vi "Master_DAQ.vi"(8 "error in (no error)":errorcluster) -> (0 "error out":errorcluster)   [LabVIEW 2018]
doc: "Reads actual data from inputs or virtual data for testing. Converts the data into an array of double precision values and sends it to the user, HostMain.vi, and the main control loop."
uses:
  Type_Def/TypeDef_LoopPeriod.ctl
  Type_Def/Type_Def NetworkStreamState.ctl
  Type_Def/Master_DataControl.ctl
  Type_Def/TypeDef_cRIODatas.ctl
  Type_Def/Type_Def IMUDatas.ctl
  Type_Def/TypeDef_BMSDatas.ctl
  Type_Def/TypeDef_BMSStatuss.ctl
  Type_Def/TypeDef FixedMotorData.ctl
  Type_Def/Type_Def Master_DataControls.ctl
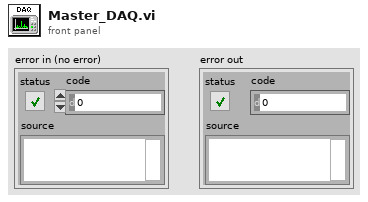
[diagram p1: front panel]
types:
  T1 = typedef "TypeDef_LoopPeriod.ctl" = cluster{"Control Period":i64, "DAQ Period":u32, "IMU Period":u32, "CAN Period":i64, "Nav Period":u32}
  T2 = typedef "Type_Def NetworkStreamState.ctl" = enum16{"Wait", "Test", "Initialize", "Read/Write", "Terminate"}
  T3 = typedef "Type_Def Master_DataControls.ctl" = cluster{"cRIO Data":T4, "IMU Data":T5, "BMS Data":T6, "Motor Data":T8}
  T4 = typedef "TypeDef_cRIODatas.ctl" = cluster{"HallEffect Right (cm)":dbl, "HallEffect Left (cm)":dbl, "Optical Sensor 1 (V)":dbl, "Optical Sensor 2 (V)":dbl, "24V Voltage  (V)":dbl, "24V Current (A)":dbl, "Contactor H1 Continuity":dbl, "Contactor L1 Continuity ":dbl, "Contactor H2 Continuity":dbl, "Contactor L2 Continuity ":dbl, "Brake PT(psig)":dbl, "Pump PT (psig)":dbl, "24V Temp   (C)":dbl, "Tank PT(psig) ":dbl, "ABS Pressure 1 (psig)":dbl, "ABS Pressure 2 (psig) ":dbl, "Displacement (ft)":dbl, "Velocity (ft/s)":dbl, "Time (ms)":dbl}
  T5 = typedef "Type_Def IMUDatas.ctl" = cluster{"x acceleration (g)":dbl, "Pressure (psia)":dbl, "Temperature (F)":dbl}
  T6 = typedef "TypeDef_BMSDatas.ctl" = cluster{"Pack 1 Max Cell\n Voltage (V)":dbl, "Pack 1 Max Cell\n ID ":dbl, "Pack 1 Min Cell \nVoltage (V)":dbl, "Pack 1 Min Cell \nID ":dbl, "Pack 1 State of Charge  (%)":dbl, "Pack 1 Average Voltage1 (V)":dbl, "Pack 1Voltage Delta (V)":dbl, "Pack 1 Current (A)":dbl, "Pack 1 Voltage (V)":dbl, "Pack 1 Max Resistance (Ohm)":dbl, "Pack 1Min Resistance (Ohm)":dbl, "Pack 1Average Resistance (Ohm)":dbl, "Pack 1Delta Resistance (Ohm)":dbl, "Pack 1 Highest Temperature(F)":dbl, "BmsStatus":T7, "Pack 2 Max Cell\n Voltage (V) ":dbl, "Pack 2 Max Cell\n ID  ":dbl, "Pack 2 Min Cell \nVoltage (V) ":dbl, "Pack 2 Min Cell \nID  ":dbl, "Pack 2 Average Voltage1 (V)":dbl, "Pack 2 Voltage Delta (V) ":dbl, "Pack 2 Current (A)":dbl, "Pack 2 Voltage (V) ":dbl, "Pack 2 State of Charge  (%) ":dbl, "Pack 2 Max Resistance (Ohm) ":dbl, "Pack 2 Min Resistance (Ohm)":dbl, "Pack 2 Average Resistance (Ohm)":dbl, "Pack 2 Delta Resistance (Ohm) ":dbl, "Pack 2 Highest Temperature(F) ":dbl}
  T7 = typedef "TypeDef_BMSStatuss.ctl" = cluster{"isFault":bool, "isolationMonitoring":bool, "isFault 2":bool, "isolationMonitoring 2":bool}
  T8 = typedef "TypeDef FixedMotorData.ctl" = cluster{" Velocity (RPM)":dbl, " MotorTemp(C)":dbl, " ControlTemp(C)":dbl, " DcLinkVolt(V)":dbl, " ErrorCode":dbl, "IsAlive":bool, "motorStatus":cluster{"isReady":bool, "isOn":bool, "isOperEn":bool, "isFault":bool, "isVoltEn":bool, "targetReached":bool, "isWarning":bool}, "motorControllerState":u16}
  T9 = typedef "Master_DataControl.ctl" = cluster{"cRIO Data":T4, "IMU Data":T5, "BMS Data":T6, "Motor Data":T8}
  T10 = cluster{"x acceleration (g)":dbl, "Pressure (psia)":dbl, "Temperature (F)":dbl}
  T11 = typedef "TypeDef_NetworkStreamState.ctl" = enum16{"Wait", "Test", "Initialize", "Read/Write", "Terminate"}
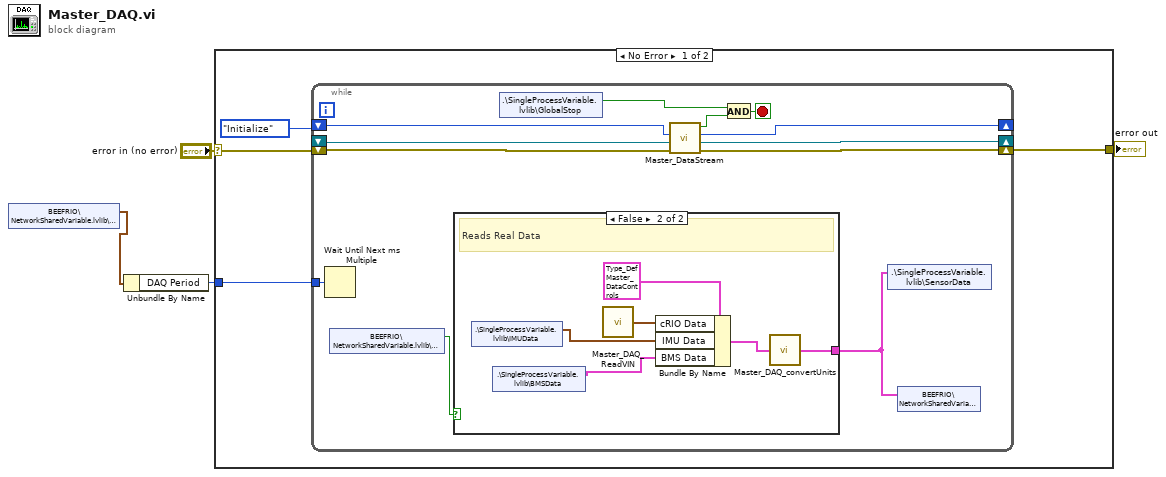
[diagram p0: block diagram]
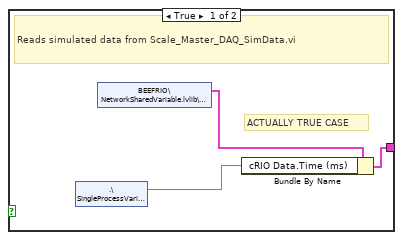
[diagram p2: hidden frame]
diagram:
  n1 = shared-variable "BEEFRIO\\NetworkSharedVariable.lvlib\\LoopPeriods"() -> (w1:T1)  [unwired: 1 in, 1 out]
  n2 = Unbundle By Name(w1) -> ("DAQ Period"=w2:u32)
  n3 = case shown="No Error" "error in (no error)" {
    selector: "error in (no error)" -> [w8 w30]
    tunnel: [w7 w30] -> w3
    tunnel: w2 -> [w6 _]
    frame No Error {
      n4 = while {
        shift-right: [w16] -> w7
        shift-left: w8 -> [w17]
        shift-right: [w20] -> _
        shift-left: _ -> [w14]
        tunnel: w6 -> [w15]
        shift-right: [w9] -> _
        shift-left: Type_Def_NetworkStreamState."Initialize" ("Enum") -> [w10]
        stop <- w19 stop-if-true
        n5 = Wait Until Next ms Multiple(millisecond multiple=w15) -> ()  [unwired: 1 out]
        n6 = shared-variable "BEEFRIO\\NetworkSharedVariable.lvlib\\SimulateData"() -> (w11:bool)  [unwired: 1 in, 1 out]
        n7 = case shown="False" w11 {
          tunnel: [w21 w24] -> w12
          frame True {
            # "ACTUALLY TRUE CASE"
            # "Reads simulated data from Scale_Master_DAQ_SimData.vi"
            n8 = shared-variable ".\\SingleProcessVariable.lvlib\\Time"() -> (w23:dbl)  [unwired: 1 in, 1 out]
            n9 = shared-variable "BEEFRIO\\NetworkSharedVariable.lvlib\\DataOverride"() -> (w22:T9)  [unwired: 1 in, 1 out]
            n10 = Bundle By Name(cluster=w22, "cRIO Data.Time (ms)"=w23) -> (w21:T9)
          }
          frame False {
            # "Reads Real Data"
            n11 = shared-variable ".\\SingleProcessVariable.lvlib\\IMUData"() -> (w26:T10)  [unwired: 1 in, 1 out]
            n12 = shared-variable ".\\SingleProcessVariable.lvlib\\BMSData"() -> (w25:T6)  [unwired: 1 in, 1 out]
            n13 = call "Master_DAQ_ReadVIN.vi"() -> ("cRIO Data"=w27:T4)  [unwired: 1 in]
            n14 = Bundle By Name(cluster=T3 {"cRIO Data"={"HallEffect Right (cm)"=0.0, "HallEffect Left (cm)"=0.0, "Optical Sensor 1 (V)"=0.0, "Optical Sensor 2 (V)"=0.0, "24V Voltage  (V)"=0.0, "24V Current (A)"=0.0, "Contactor H1 Continuity"=0.0, "Contactor L1 Continuity "=0.0, "Contactor H2 Continuity"=0.0, "Contactor L2 Continuity "=0.0, "Brake PT(psig)"=0.0, "Pump PT (psig)"=0.0, "24V Temp   (C)"=0.0, "Tank PT(psig) "=0.0, "ABS Pressure 1 (psig)"=0.0, "ABS Pressure 2 (psig) "=0.0, "Displacement (ft)"=0.0, "Velocity (ft/s)"=0.0, "Time (ms)"=0.0}, "IMU Data"={"x acceleration (g)"=0.0, "Pressure (psia)"=0.0, "Temperature (F)"=0.0}, "BMS Data"={"Pack 1 Max Cell\n Voltage (V)"=0.0, "Pack 1 Max Cell\n ID "=0.0, "Pack 1 Min Cell \nVoltage (V)"=0.0, "Pack 1 Min Cell \nID "=0.0, "Pack 1 State of Charge  (%)"=0.0, "Pack 1 Average Voltage1 (V)"=0.0, "Pack 1Voltage Delta (V)"=0.0, "Pack 1 Current (A)"=0.0, "Pack 1 Voltage (V)"=0.0, "Pack 1 Max Resistance (Ohm)"=0.0, "Pack 1Min Resistance (Ohm)"=0.0, "Pack 1Average Resistance (Ohm)"=0.0, "Pack 1Delta Resistance (Ohm)"=0.0, "Pack 1 Highest Temperature(F)"=0.0, "BmsStatus"={"isFault"=FALSE, "isolationMonitoring"=FALSE, "isFault 2"=FALSE, "isolationMonitoring 2"=FALSE}, "Pack 2 Max Cell\n Voltage (V) "=0.0, "Pack 2 Max Cell\n ID  "=0.0, "Pack 2 Min Cell \nVoltage (V) "=0.0, "Pack 2 Min Cell \nID  "=0.0, "Pack 2 Average Voltage1 (V)"=0.0, "Pack 2 Voltage Delta (V) "=0.0, "Pack 2 Current (A)"=0.0, "Pack 2 Voltage (V) "=0.0, "Pack 2 State of Charge  (%) "=0.0, "Pack 2 Max Resistance (Ohm) "=0.0, "Pack 2 Min Resistance (Ohm)"=0.0, "Pack 2 Average Resistance (Ohm)"=0.0, "Pack 2 Delta Resistance (Ohm) "=0.0, "Pack 2 Highest Temperature(F) "=0.0}, "Motor Data"={" Velocity (RPM)"=0.0, " MotorTemp(C)"=0.0, " ControlTemp(C)"=0.0, " DcLinkVolt(V)"=0.0, " ErrorCode"=0.0, "IsAlive"=FALSE, "motorStatus"={"isReady"=FALSE, "isOn"=FALSE, "isOperEn"=FALSE, "isFault"=FALSE, "isVoltEn"=FALSE, "targetReached"=FALSE, "isWarning"=FALSE}, "motorControllerState"=1}}, "cRIO Data"=w27, "IMU Data"=w26, "BMS Data"=w25) -> (w28:T3)
            n15 = call "Master_DAQ_convertUnits.vi"("Data Control In"=w28) -> ("Data Out"=w24:T3)
          }
        }
        n16 = shared-variable ".\\SingleProcessVariable.lvlib\\GlobalStop"() -> (w13:bool)  [unwired: 1 in, 1 out]
        n17 = call "Master_DataStream.vi"("error in"=w17, "reader name in"=w14, "Enum in"=w10) -> ("error out"=w16:errorcluster, "reader name out"=w20:refnum<k21>, "Enum out"=w9:T11, "Boolean"=w18:bool)  [unwired: 5 in]
        n18 = And(x=w13, y=w18) -> (x .and. y?=w19:bool)
        n19 = shared-variable ".\\SingleProcessVariable.lvlib\\SensorData"(w12) -> ()  [unwired: 1 in, 1 out]
        n20 = shared-variable "BEEFRIO\\NetworkSharedVariable.lvlib\\AllData"(w12) -> ()  [unwired: 1 in, 1 out]
      }
    }
    frame Error {
    }
  }
  "error out" <- w3
